vi "Set Output Node Linkage.vi"(7 "Add?":bool, 8 "error in":errorcluster, 11 "Section Ref in":T1 format="%.0x") -> (0 "error out":errorcluster, 3 "Item Ref out":T1 format="%.0x")   [LabVIEW 2019, in "Control Addon Shared.lvlib"]
uses:
  Control Addon Shared.lvlib
  <vilib>/NI VeriStand/Custom Device API/Custom Device Item Ref.ctl
  NationalInstruments.VeriStand.SystemStorage
  Constants.vi
  <vilib>/NI VeriStand/Custom Device Tools/Custom Device Utility Library/NI VeriStand - Search for Item by GUID.vi
  <vilib>/NI VeriStand/Custom Device API/Get Item Property (Dependent Node Pointer).vi
  <vilib>/NI VeriStand/Custom Device API/Custom Device API.lvlib
  <vilib>/NI VeriStand/Custom Device Tools/Custom Device Utility Library/Custom Device Utility Library.lvlib
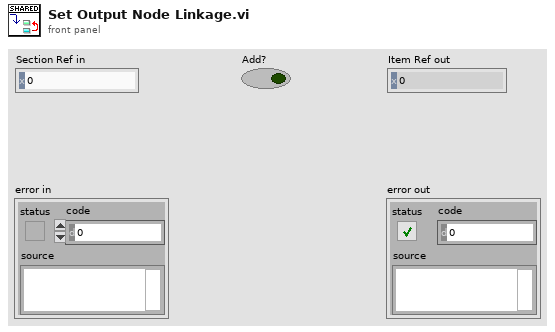
[diagram p1: front panel]
types:
  T1 = typedef "Custom Device API.lvlib/Custom Device Item Ref.ctl" = u64
  T2 = typedef "Custom Device API.lvlib/Custom Device Pointer.ctl" = refnum<k24>
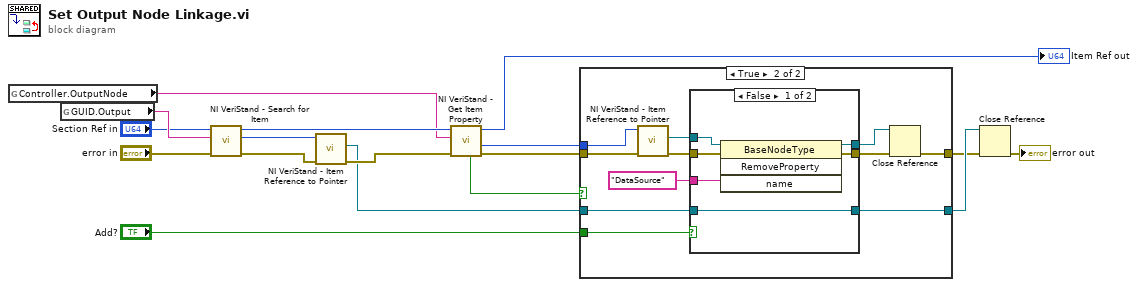
[diagram p0: block diagram]
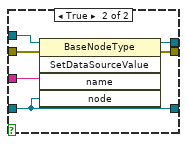
[diagram p3: hidden frame]
diagram:
  n1 = global read "Constants.vi" "Controller.OutputNode"() -> (w3:string)
  n2 = global read "Constants.vi" "GUID.Output"() -> (w15:string)
  n3 = call-poly <vilib>:"NI VeriStand - Search for Item.vi"("error in"="error in", "Item GUID"=w15, "Section Ref in"="Section Ref in") -> ("error out"=w12:errorcluster, "Item Ref"=w13:T1, "Section Ref out"=w14:T1)  [unwired: 5 in, 1 out]
  n4 = call <vilib>:"NI VeriStand - Item Reference to Pointer.vi"("error in (no error)"=w12, "Item Ref in"=w13) -> ("error out"=w11:errorcluster, "Node Pointer"=w10:T2)  [unwired: 6 in, 2 out]
  n5 = call-poly <vilib>:"NI VeriStand - Get Item Property.vi"("error in (no error)"=w11, "Property Name"=w3, "Item Ref in"=w14) -> ("error out"=w16:errorcluster, "Dependent Node Ref"=w17:T1, "Item Ref out"=→"Item Ref out":T1, "Found"=w2:bool)  [unwired: 5 in]
  n6 = case shown="True" w2 {
    tunnel: w17 -> [_ w30]
    tunnel: w16 -> [w18 w29]
    tunnel: w10 -> [w19 w25]
    tunnel: [w18 w22] -> w1
    tunnel: [w19 w24] -> w9
    tunnel: "Add?" -> [_ w23]
    frame False {
    }
    frame True {
      n7 = call <vilib>:"NI VeriStand - Item Reference to Pointer.vi"("error in (no error)"=w29, "Item Ref in"=w30) -> ("error out"=w28:errorcluster, "Node Pointer"=w27:T2)  [unwired: 6 in, 2 out]
      n8 = case shown="False" w23 {
        tunnel: [w33 w42] -> w20
        tunnel: [w34 w41] -> w21
        tunnel: w25 -> [w31 w37]
        tunnel: w28 -> [w35 w40]
        tunnel: w27 -> [w36 w39]
        tunnel: "DataSource" ("name") -> [w32 w38]
        tunnel: [w31 w37] -> w24
        frame False {
          n9 = invoke class="BaseNodeType" method="RemoveProperty"(reference=w36, error in=w35, "name"=w32) -> (reference out=w33:T2, error out=w34:errorcluster)  [unwired: 1 in, 2 out]
        }
        frame True {
          n10 = invoke class="BaseNodeType" method="SetDataSourceValue"(reference=w39, error in=w40, "name"=w38, "node"=w37) -> (reference out=w42:T2, error out=w41:errorcluster)  [unwired: 1 in, 3 out]
        }
      }
      n11 = Close Reference(reference=w20, error in (no error)=w21) -> (error out=w22:errorcluster)
    }
  }
  n12 = Close Reference(reference=w9, error in (no error)=w1) -> (error out=→"error out":errorcluster)
